vi "Find Project Square Paths.vi"(11 "Project":refnum<vi>) -> (0 "error out":errorcluster, 2 "Square Run VIs":path[](array[path]), 3 "Base Square":path)   [LabVIEW 2020]
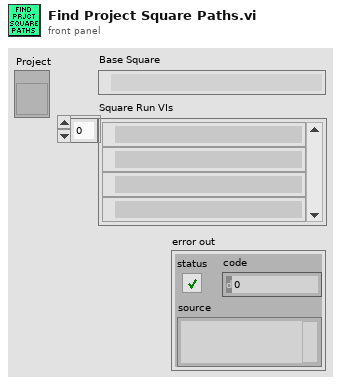
[diagram p1: front panel]
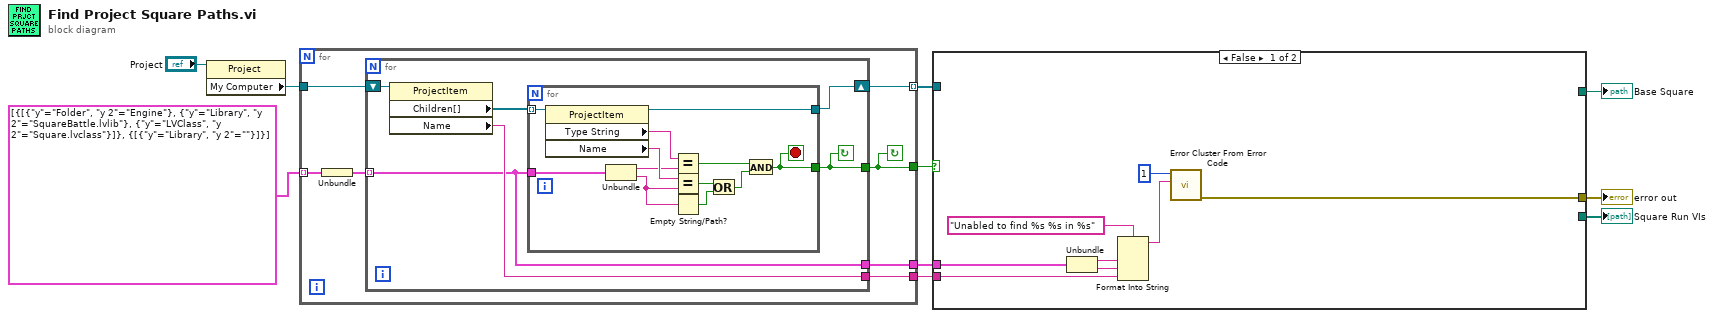
[diagram p0: block diagram]
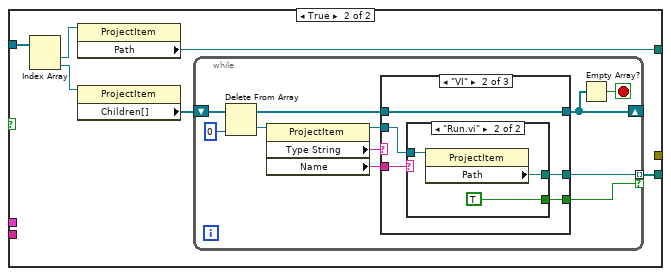
[diagram p2: hidden frame]
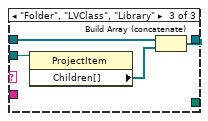
[diagram p5: hidden frame]
diagram:
  n1 = property class="Project"(reference="Project") -> ("My Computer"=w10:refnum<vi>)  [unwired: 1 in, 2 out]
  n2 = for {
    tunnel: w10 -> [w17]
    tunnel: cluster{cluster{"y":string, "y 2":string}[]}[] [{[{"y"="Folder", "y 2"="Engine"}, {"y"="Library", "y 2"="SquareBattle.lvlib"}, {"y"="LVClass", "y 2"="Square.lvclass"}]}, {[{"y"="Library", "y 2"=""}]}] -> [w16] mode=indexing
    tunnel: [w14] -> w8 mode=indexing
    tunnel: [w13] -> w7
    tunnel: [w12] -> w5
    tunnel: [w11] -> w6
    stop <- w13 continue-if-true
    n3 = Unbundle(w16) -> (w15:cluster{"y":string, "y 2":string}[])
    n4 = for {
      shift-right: [w21] -> w14
      shift-left: w17 -> [w23]
      tunnel: w15 -> [w18] mode=indexing
      tunnel: [w20] -> w13
      tunnel: [w19] -> w12
      tunnel: [w18] -> w11
      stop <- w20 continue-if-true
      n5 = property class="ProjectItem"(reference=w23) -> ("Children[]"=w22:refnum<vi>[], "Name"=w19:string)  [unwired: 1 in, 2 out]
      n6 = for {
        tunnel: w22 -> [w35] mode=indexing
        tunnel: [w33] -> w21
        tunnel: w18 -> [w29]
        tunnel: [w27] -> w20
        stop <- w27 stop-if-true
        n7 = property class="ProjectItem"(reference=w35) -> (reference out=w33:refnum<vi>, "Type String"=w34:string, "Name"=w32:string)  [unwired: 1 in, 1 out]
        n8 = Unbundle(w29) -> ("y"=w28:string, "y 2"=w26:string)
        n9 = Equal?(x=w34, y=w28) -> (x = y?=w31:bool)
        n10 = Equal?(x=w32, y=w26) -> (x = y?=w30:bool)
        n11 = Empty String/Path?(string/path=w26) -> (empty?=w24:bool)
        n12 = Or(x=w30, y=w24) -> (x .or. y?=w25:bool)
        n13 = And(x=w31, y=w25) -> (x .and. y?=w27:bool)
      }
    }
  }
  n14 = case shown="False" w7 {
    tunnel: w8 -> [_ w49]
    tunnel: w6 -> [w41 _]
    tunnel: w5 -> [w38 _]
    tunnel: [w36 _] -> w4
    tunnel: [_ w47] -> w3
    tunnel: [_ w44] -> w2
    frame False {
      n15 = Unbundle(w41) -> ("y"=w40:string, "y 2"=w39:string)
      n16 = Format Into String(format string="Unabled to find %s %s in %s", w40, w39, w38) -> (resulting string=w37:string)  [unwired: 2 in, 1 out]
      n17 = call <vilib>:"Error Cluster From Error Code.vi"("error message (\"\")"=w37, "error code (0)"=1) -> ("error out"=w36:errorcluster)  [unwired: 7 in]
    }
    frame True {
      n18 = Index Array(array=w49) -> (element #1=w48:refnum<vi>, element #2=w46:refnum<vi>)  [unwired: 2 in]
      n19 = property class="ProjectItem"(reference=w48) -> ("Path"=w47:path)  [unwired: 1 in, 2 out]
      n20 = property class="ProjectItem"(reference=w46) -> ("Children[]"=w45:refnum<vi>[])  [unwired: 1 in, 2 out]
      n21 = while {
        shift-right: [w54] -> _
        shift-left: w45 -> [w60]
        tunnel: [w51] -> w44 mode=indexing if=w50
        stop <- w53 stop-if-true
        n22 = Delete From Array(array=w60, index=0) -> (deleted portion=w58:refnum<vi>, array with subset deleted=w56:refnum<vi>[])  [unwired: 1 in]
        n23 = property class="ProjectItem"(reference=w58) -> (reference out=w55:refnum<vi>, "Type String"=w57:string, "Name"=w52:string)  [unwired: 1 in, 1 out]
        n24 = case shown="\"VI\"" w57 {
          tunnel: w56 -> [w61 w65 w72]
          tunnel: [w61 w65 w70] -> w54
          tunnel: w55 -> [_ w64 w73]
          tunnel: w52 -> [_ w66 _]
          tunnel: [_ w63 _] -> w51
          tunnel: [_ w62 _] -> w50
          frame Default {
          }
          frame "VI" {
            n25 = case shown="\"Run.vi\"" w66 {
              tunnel: w64 -> [_ w69]
              tunnel: [_ w68] -> w63
              tunnel: [_ TRUE] -> w62
              frame "False", Default {
              }
              frame "Run.vi" {
                n26 = property class="ProjectItem"(reference=w69) -> ("Path"=w68:path)  [unwired: 1 in, 2 out]
              }
            }
          }
          frame "Folder", "LVClass", "Library" {
            n27 = property class="ProjectItem"(reference=w73) -> ("Children[]"=w71:refnum<vi>[])  [unwired: 1 in, 2 out]
            n28 = Build Array (concatenate)(w72, w71) -> (w70:refnum<vi>[])
          }
        }
        n29 = Empty Array?(array=w54) -> (empty?=w53:bool)
      }
    }
  }
  "Base Square" <- w3
  "error out" <- w4
  "Square Run VIs" <- w2
